vi "tsa_NFFT.vi"(8 "nfft":i32, 11 "X":dbl[](array[numeric])) -> (0 "error":i32, 3 "FFT {X}":cdb[](array[numeric]))   [LabVIEW 2020, in "NI_AALPro.lvlib"]
uses:
  <vilib>/Analysis/NI_AALPro.lvlib
  <vilib>/Analysis/2dsp.llb/Real FFT.vi
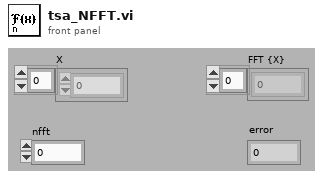
[diagram p1: front panel]
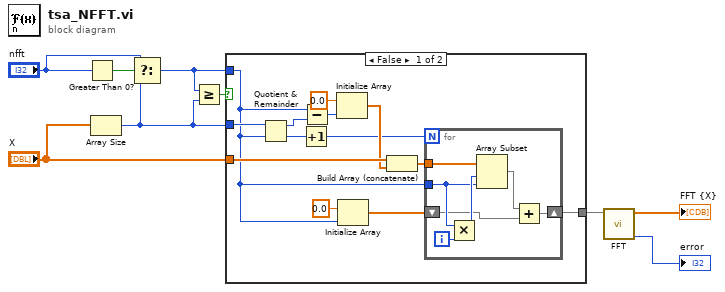
[diagram p0: block diagram]
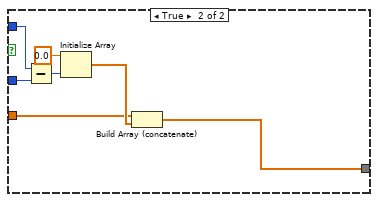
[diagram p2: hidden frame]
diagram:
  n1 = Greater Than 0?(x="nfft") -> (x > 0?=w4:bool)
  n2 = Array Size(array="X") -> (size(s)=w5:i32)
  n3 = Select(t="nfft", s=w4, f=w5) -> (s? t:f=w7:i32)
  n4 = Greater Or Equal?(x=w7, y=w5) -> (x >= y?=w2:bool)
  n5 = case shown="False" w2 {
    tunnel: w7 -> [w12 w35]
    tunnel: w5 -> [w22 w36]
    tunnel: "X" -> [w17 w31]
    tunnel: [w10 w30] -> w3
    frame False {
      n6 = Quotient & Remainder(x=w22, y=w12) -> (x-y*floor(x/y)=w20:i32, floor(x/y)=w21:i32)
      n7 = Increment(x=w21) -> (x+1=w15:i32)
      n8 = Subtract(x=w12, y=w20) -> (x-y=w19:i32)
      n9 = Initialize Array(0.0 ("element"), w19) -> (w16:dbl[])
      n10 = Initialize Array(0.0 ("element"), w12) -> (w11:dbl[])
      n11 = Build Array (concatenate)(w17, w16) -> (w14:dbl[])
      n12 = for {
        N: w15 -> [_]
        tunnel: w14 -> [w29]
        shift-right: [w25] -> w10
        shift-left: w11 -> [w24]
        tunnel: w12 -> [w26]
        i -> [w28]
        n13 = Multiply(x=w26, y=w28) -> (x*y=w27:i32)
        n14 = Array Subset(array=w29, index=w27, length=w26) -> (w23:dbl[])
        n15 = Add(x=w23, y=w24) -> (x+y=w25:dbl[])
      }
    }
    frame True {
      n16 = Subtract(x=w35, y=w36) -> (x-y=w34:i32)
      n17 = Initialize Array(0.0 ("element"), w34) -> (w32:dbl[])
      n18 = Build Array (concatenate)(w31, w32) -> (w30:dbl[])
    }
  }
  n19 = call-poly <vilib>:"FFT.vi"("X"=w3) -> ("error"=→"error":i32, "FFT {X}"=→"FFT {X}":cdb[])  [unwired: 9 in]
